vi "Test ReadingWriting to SoftwareSerial.vi"   [LabVIEW 2014, in "Arduino SoftwareSerial Wrapper.lvlib"]
uses:
  <vilib>/Aledyne-TSXperts/Arduino Compatible Compiler for LabVIEW/addons/Arduino SoftwareSerial Wrapper/Arduino SoftwareSerial Wrapper.lvlib
  <vilib>/Aledyne-TSXperts/Arduino Compatible Compiler for LabVIEW/Code Generator/Arduino APIs/Serial/Serial Settings.ctl
  <vilib>/Aledyne-TSXperts/Arduino Compatible Compiler for LabVIEW/Arduino Compatible Compiler for LabVIEW.lvlib
types:
  T1 = typedef "Arduino Compatible Compiler for LabVIEW.lvlib/Serial Settings.ctl" = u16
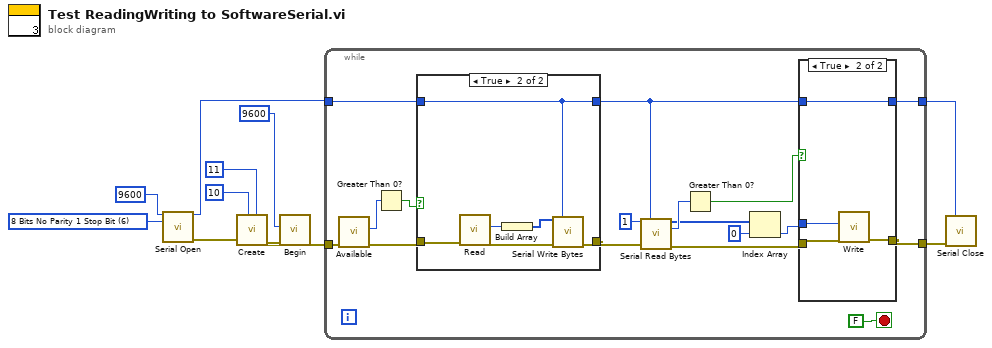
[diagram p0: block diagram]
diagram:
  w10 = T1 6 items=["5 Bits No Parity 1 Stop Bit"=0, "6 Bits No Parity 1 Stop Bit"=2, "7 Bits No Parity 1 Stop Bit"=4, "8 Bits No Parity 1 Stop Bit"=6, "5 Bits No Parity 2 Stop Bits"=8, "6 Bits No Parity 2 Stop Bits"=10, "7 Bits No Parity 2 Stop Bits"=12, "8 Bits No Parity 2 Stop Bits"=14, "5 Bits Even Parity 1 Stop Bits"=32, "6 Bits Even Parity 1 Stop Bits"=34, "7 Bits Even Parity 1 Stop Bits"=36, "8 Bits Even Parity 1 Stop Bits"=38, "5 Bits Even Parity 2 Stop Bits"=40, "6 Bits Even Parity 2 Stop Bits"=42, "7 Bits Even Parity 2 Stop Bits"=44, "8 Bits Even Parity 2 Stop Bits"=46, "5 Bits Odd Parity 1 Stop Bits"=48, "6 Bits Odd Parity 1 Stop Bits"=50, "7 Bits Odd Parity 1 Stop Bits"=52, "8 Bits Odd Parity 1 Stop Bits"=54, "5 Bits Odd Parity 2 Stop Bits"=56, "6 Bits Odd Parity 2 Stop Bits"=58, "7 Bits Odd Parity 2 Stop Bits"=60, "8 Bits Odd Parity 2 Stop Bits"=62] ("Serial Settings")
  n1 = call <vilib>:"Serial Open.vi"("Speed"=u32 9600, "Serial Settings"=w10) -> ("Instance"=w8:u8, "error out"=w9:errorcluster)  [unwired: 12 in]
  n2 = call <vilib>:"Create.vi"("arduino TX pin"=u8 11 ("TX pin"), "arduino RX pin"=u8 10 ("RX pin"), "Error In"=w9) -> ("Error Out"=w7:errorcluster)  [unwired: 8 in]
  n3 = call <vilib>:"Begin.vi"("Error In"=w7, "Baudrate"=u16 9600) -> ("Error Out"=w6:errorcluster)  [unwired: 8 in]
  n4 = while {
    tunnel: w6 -> [w26]
    tunnel: w8 -> [w27]
    tunnel: [w21] -> w1
    tunnel: [w23] -> w4
    stop <- FALSE stop-if-true
    n5 = call <vilib>:"Available.vi"("Error In"=w26) -> ("Error Out"=w18:errorcluster, "Bytes to read"=w17:u16)  [unwired: 9 in]
    n6 = Greater Than 0?(x=w17) -> (x > 0?=w16:bool)
    n7 = case shown="True" w16 {
      tunnel: w18 -> [w30 w36]
      tunnel: w27 -> [w29 w35]
      tunnel: [w30 w32] -> w25
      tunnel: [w29 w35] -> w24
      frame False {
      }
      frame True {
        n8 = call <vilib>:"Read.vi"("Error In"=w36) -> ("Error Out"=w31:errorcluster, "Output char"=w34:u8)  [unwired: 9 in]
        n9 = Build Array(w34) -> (w33:u8[])
        n10 = call <vilib>:"Serial Write Bytes.vi"("Data"=w33, "Instance"=w35, "error in (no error)"=w31) -> ("error out"=w32:errorcluster)  [unwired: 12 in]
      }
    }
    n11 = call <vilib>:"Serial Read Bytes.vi"("Length"=1, "Instance"=w24, "error in (no error)"=w25) -> ("Data"=w14:u8[], "Bytes Read"=w15:u16, "error out"=w20:errorcluster)  [unwired: 10 in]
    n12 = Greater Than 0?(x=w15) -> (x > 0?=w22:bool)
    n13 = Index Array(array=w14, index=0) -> (element=w12:u8)
    n14 = case shown="True" w22 {
      tunnel: w24 -> [w38 w41]
      tunnel: [w38 w41] -> w23
      tunnel: [w37 w42] -> w21
      tunnel: w20 -> [w37 w40]
      tunnel: w12 -> [_ w39]
      frame False {
      }
      frame True {
        n15 = call <vilib>:"Write.vi"("Error In"=w40, "Char to write"=w39) -> ("Error Out"=w42:errorcluster)  [unwired: 9 in]
      }
    }
  }
  n16 = call <vilib>:"Serial Close.vi"("Instance"=w4, "error in (no error)"=w1) -> ()  [unwired: 13 in, 1 out]
